vi "global_all_rt_loop_stop.vi"() -> ()   [LabVIEW 2015]
panel:
  in  "All RT Loop Stop":bool caption="全部RT循环停止"
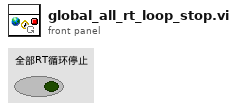
[diagram p1: front panel]
diagram:
